vi "Build Proto.vi"(6 "Include Paths (None)":path[](array[path]), 8 "error in (no error)":errorcluster, 10 "Output Folder":path=path "C:/dev/proto/hello/lv", 11 ".proto Path":path=path "C:/dev/proto/hello/hello.proto") -> (0 "error out":errorcluster, 3 "LV-Protoc out":refnum<class "LV-Protoc.lvclass">)   [LabVIEW 2020, in "LV-Protoc.lvlib" / "LV-Protoc.lvclass"]
uses:
  LV-Protoc.lvclass
  ProtoParser/ProtoParser.lvclass
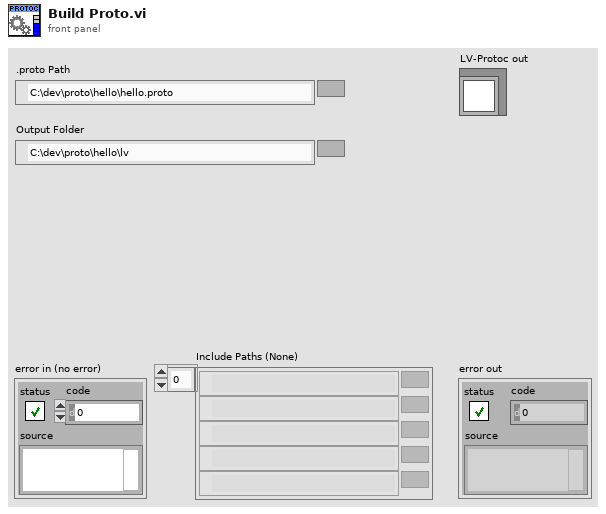
[diagram p1: front panel]
types:
  T1 = typedef "LV-Proto.lvlib/Message.ctl" = cluster{"Name":string, "Fields":T2[], "Reserved Numbers":u32[], "Reserved Names":string[]}
  T2 = typedef "LV-Proto.lvlib/Field.ctl" = cluster{"Name":string, "Number":u32, "Optional":bool, "Repeated":bool, "Type":T3, "Key Type":T3, "Value Type":T3}
  T3 = typedef "LV-Proto.lvlib/Type.ctl" = cluster{"Type":T4, "Subtype":string}
  T4 = typedef "LV-Proto.lvlib/Proto Type.ctl" = enum16{"UNKNOWN", "double", "float", "int32", "int64", "uint32", "uint64", "sint32", "sint64", "fixed32", "fixed64", "sfixed32", "sfixed64", "bool", "string", "bytes", "enum", "map", "message"}
  T5 = typedef "LV-Proto.lvlib/Enumeration.ctl" = cluster{"Name":string, "Values":T6[], "Reserved Numbers":u32[], "Reserved Names":string[]}
  T6 = typedef "LV-Proto.lvlib/Enum Value.ctl" = cluster{"Name":string, "Value":i32}
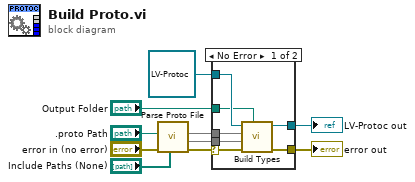
[diagram p0: block diagram]
diagram:
  n1 = call "Parse Proto File.vi"("Include Paths (None)"="Include Paths (None)", "error in (no error)"="error in (no error)", ".proto Path"=".proto Path") -> ("error out"=w7:errorcluster, "Messages"=w6:map{string, T1}, "Enumerations"=w5:map{string, T5})  [unwired: 5 in, 1 out]
  n2 = case shown="No Error" w7 {
    selector: w7 -> [w17 w18]
    tunnel: w6 -> [w16 _]
    tunnel: w5 -> [w15 _]
    tunnel: "Output Folder" -> [w13 _]
    tunnel: refnum<class "LV-Protoc.lvclass"> refnum ("LV-Protoc in") -> [w14 w19]
    tunnel: [w12 w18] -> w2
    tunnel: [w11 w19] -> w1
    frame No Error {
      n3 = call "Build Types.vi"("Output Folder"=w13, "error in (no error)"=w17, "Messages"=w16, "Enumerations"=w15, "LV-Protoc in"=w14) -> ("error out"=w12:errorcluster, "LV-Protoc out"=w11:refnum<class "LV-Protoc.lvclass">)  [unwired: 5 in]
    }
    frame Error {
    }
  }
  "error out" <- w2
  "LV-Protoc out" <- w1
